vi "Text Description.vi"(11 "Translator in":refnum<class "Translator.lvclass">) -> (2 "Description":string, 3 "Translator out":refnum<class "Translator.lvclass">)   [LabVIEW 2011, in "Messenging.lvlib" / "Translator.lvclass"]
uses:
  Translator.lvclass
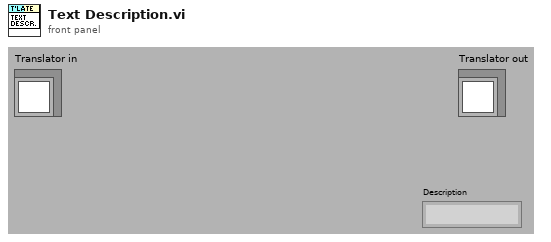
[diagram p1: front panel]
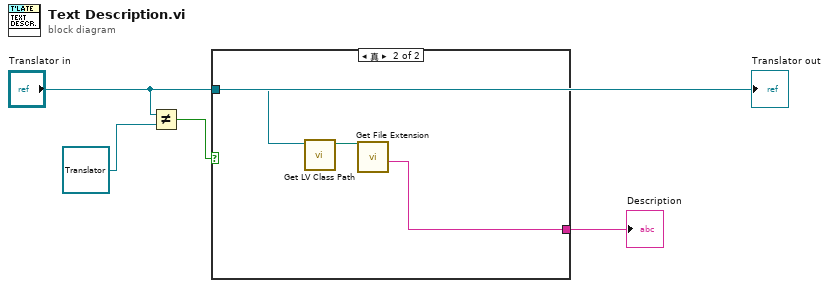
[diagram p0: block diagram]
diagram:
  n1 = Not Equal?(x="Translator in", y=refnum<class "Translator.lvclass"> refnum ("Translator in")) -> (x != y?=w2:bool)
  n2 = case shown="真" w2 {
    tunnel: [_ w6] -> w4
    tunnel: "Translator in" -> [_ w5]
    frame False {
    }
    frame True {
      n3 = call <vilib>:"Get LV Class Path.vi"("object"=w5) -> ("class path"=w7:path)  [unwired: 1 in, 9 out]
      n4 = call <vilib>:"Get File Extension.vi"("file"=w7) -> ("filename without extension"=w6:string)  [unwired: 1 in, 9 out]
    }
  }
  "Description" <- w4
  "Translator out" <- "Translator in"
